vi "MRTAnIntoPWM.vi"(10 "An In":dbl) -> (2 "PWM Out":dbl)   [LabVIEW 2009]
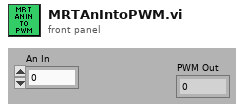
[diagram p1: front panel]
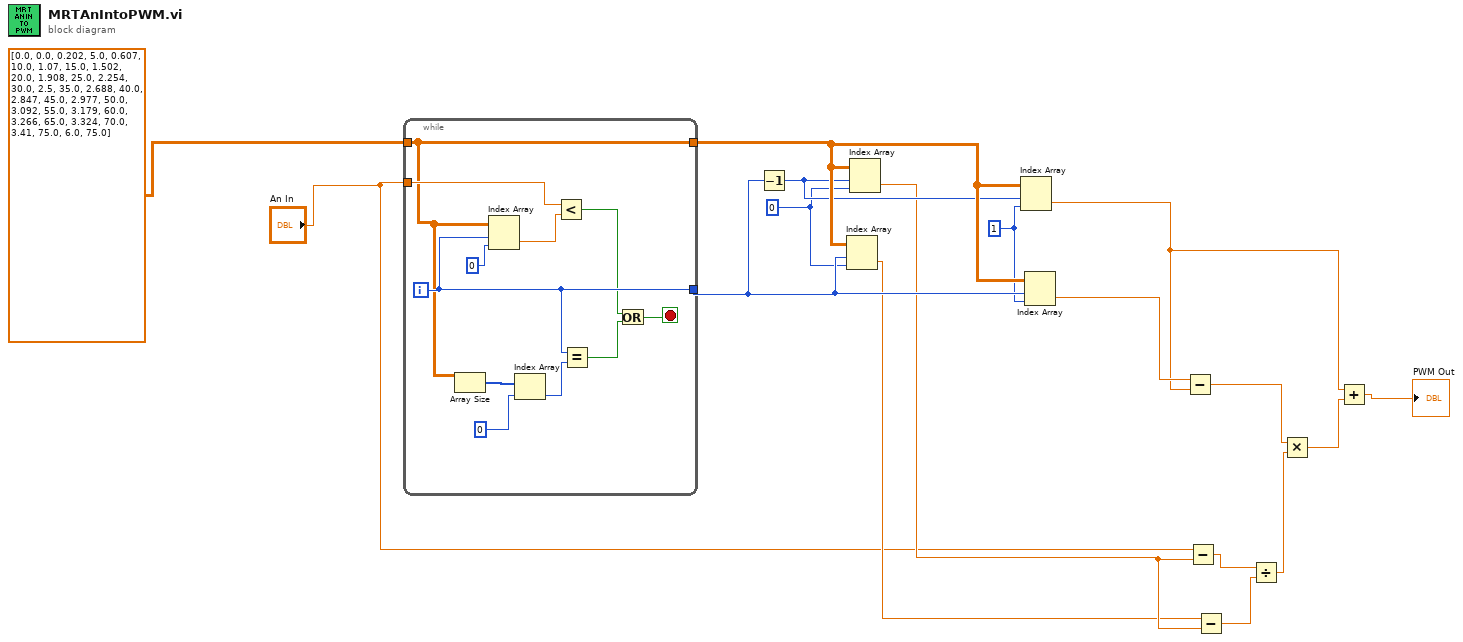
[diagram p0: block diagram]
diagram:
  w12 = 1
  w13 = 0
  n1 = while {
    tunnel: dbl[][] [[0.0, 0.0], [0.202, 5.0], [0.607, 10.0], [1.07, 15.0], [1.502, 20.0], [1.908, 25.0], [2.254, 30.0], [2.5, 35.0], [2.688, 40.0], [2.847, 45.0], [2.977, 50.0], [3.092, 55.0], [3.179, 60.0], [3.266, 65.0], [3.324, 70.0], [3.41, 75.0], [6.0, 75.0]] -> [w20]
    tunnel: [w20] -> w16
    tunnel: [w25] -> w14
    tunnel: "An In" -> [w21]
    i -> [w25]
    stop <- w24 stop-if-true
    n2 = Array Size(array=w20) -> (size(s)=w26:i32[])
    n3 = Index Array(array=w20, index (row)=w25, index (col)=0) -> (element=w27:dbl)
    n4 = Index Array(array=w26, index=0) -> (element=w19:i32)
    n5 = Less?(x=w21, y=w27) -> (x < y?=w23:bool)
    n6 = Equal?(x=w25, y=w19) -> (x = y?=w22:bool)
    n7 = Or(x=w23, y=w22) -> (x .or. y?=w24:bool)
  }
  n8 = Decrement(x=w14) -> (x-1=w15:i32)
  n9 = Index Array(array=w16, index (row)=w14, index (col)=w13) -> (element=w9:dbl)
  n10 = Index Array(array=w16, index (row)=w15, index (col)=w13) -> (element=w10:dbl)
  n11 = Index Array(array=w16, index (row)=w15, index (col)=w12) -> (element=w3:dbl)
  n12 = Index Array(array=w16, index (row)=w14, index (col)=w12) -> (element=w8:dbl)
  n13 = Subtract(x=w8, y=w3) -> (x-y=w5:dbl)
  n14 = Subtract(x="An In", y=w10) -> (x-y=w11:dbl)
  n15 = Subtract(x=w9, y=w10) -> (x-y=w7:dbl)
  n16 = Divide(x=w11, y=w7) -> (x/y=w6:dbl)
  n17 = Multiply(x=w5, y=w6) -> (x*y=w4:dbl)
  n18 = Add(x=w3, y=w4) -> (x+y=→"PWM Out":dbl)
